vi "Data To PDF.vi"(7 "Language":T1, 8 "error in":errorcluster, 11 "Inputs":T2) -> (0 "error out":errorcluster)   [LabVIEW 2016]
doc: "This VI inputs a cluster of string data, places the data into the correct cells on the cert template, then creates a PDF from the cert template."
uses:
  Controls/Language Control.ctl
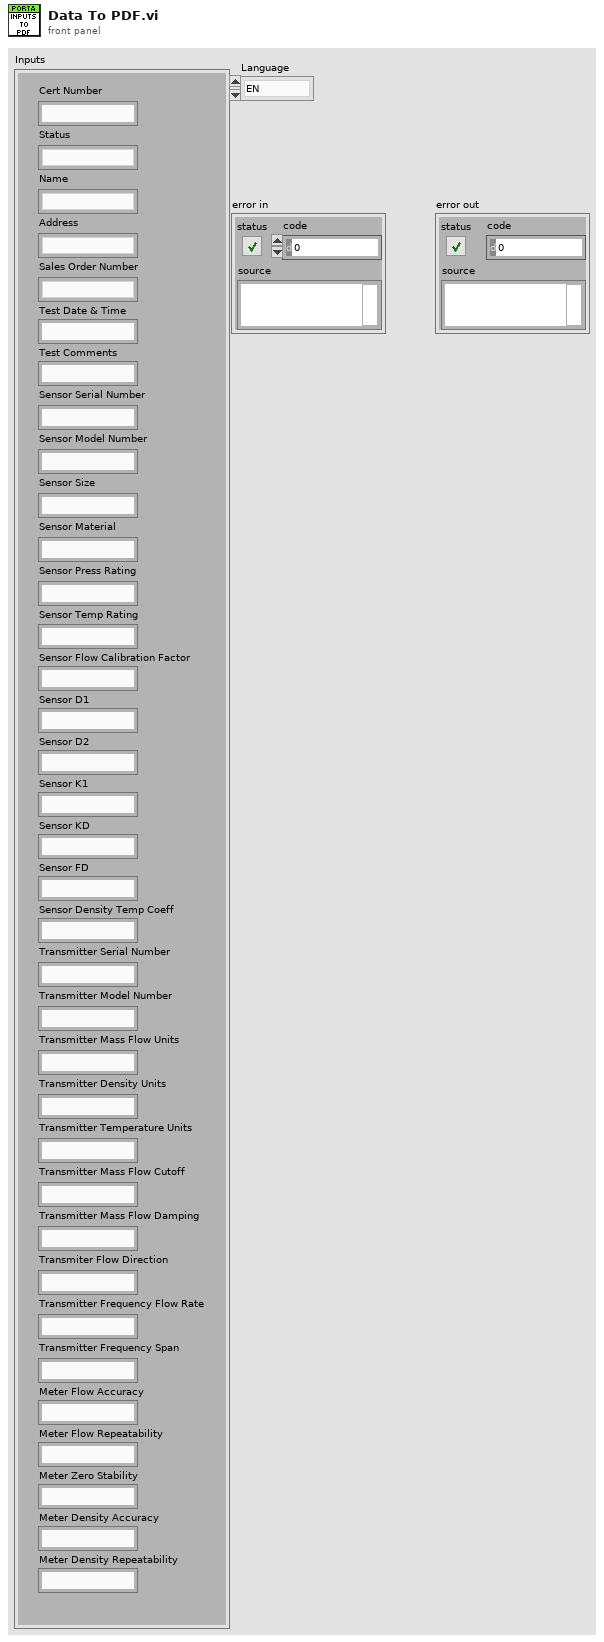
[diagram p1: front panel]
types:
  T1 = typedef "Language Control.ctl" = enum16{"EN", "ES", "FR", "RU"}
  T2 = cluster{"Cert Number":string, "Status":string, "Name":string, "Address":string, "Sales Order Number":string, "Test Date & Time":string, "Test Comments":string, "Sensor Serial Number":string, "Sensor Model Number":string, "Sensor Size":string, "Sensor Material":string, "Sensor Press Rating":string, "Sensor Temp Rating":string, "Sensor Flow Calibration Factor":string, "Sensor D1":string, "Sensor D2":string, "Sensor K1":string, "Sensor KD":string, "Sensor FD":string, "Sensor Density Temp Coeff":string, "Transmitter Serial Number":string, "Transmitter Model Number":string, "Transmitter Mass Flow Units":string, "Transmitter Density Units":string, "Transmitter Temperature Units":string, "Transmitter Mass Flow Cutoff":string, "Transmitter Mass Flow Damping":string, "Transmiter Flow Direction":string, "Transmitter Frequency Flow Rate":string, "Transmitter Frequency Span":string, "Meter Flow Accuracy":string, "Meter Flow Repeatability":string, "Meter Zero Stability":string, "Meter Density Accuracy":string, "Meter Density Repeatability":string}
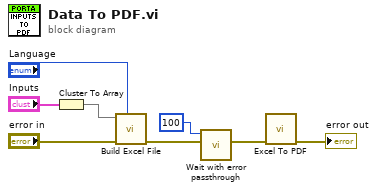
[diagram p0: block diagram]
diagram:
  n1 = Cluster To Array(cluster="Inputs") -> (array=w7:string[])
  n2 = call "Build Excel File.vi"("Gas"="Language", "error in"="error in", "Information"=w7) -> ("error out"=w4:errorcluster)  [unwired: 5 in, 3 out]
  n3 = call "Wait with error passthrough.vi"("error in"=w4, "milliseconds to wait"=u32 100) -> ("error out"=w3:errorcluster)  [unwired: 9 in]
  n4 = call "Excel To PDF.vi"("error in"=w3) -> ("error out"=→"error out":errorcluster)  [unwired: 10 in]
